vi "Read Control Height.vi"(8 "error in":errorcluster, 11 "Control in":refnum<vi>) -> (0 "error out":errorcluster, 2 "Height":u32, 3 "Control":refnum<vi>)   [LabVIEW 2020, in "VolatusGUIEditorCore.lvlib"]
uses:
  VolatusGUIEditorCore.lvlib
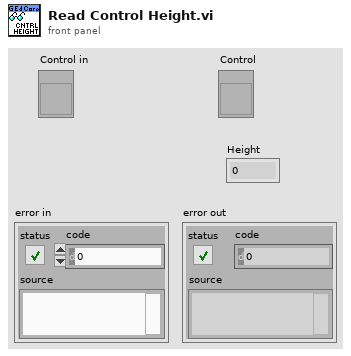
[diagram p1: front panel]
types:
  T1 = typedef "LVRectTypeDef.ctl" = cluster{"Left":i16, "Top":i16, "Right":i16, "Bottom":i16}
  T2 = typedef "LVBoundsTypeDef.ctl" = cluster{"Width":u32, "Height":u32}
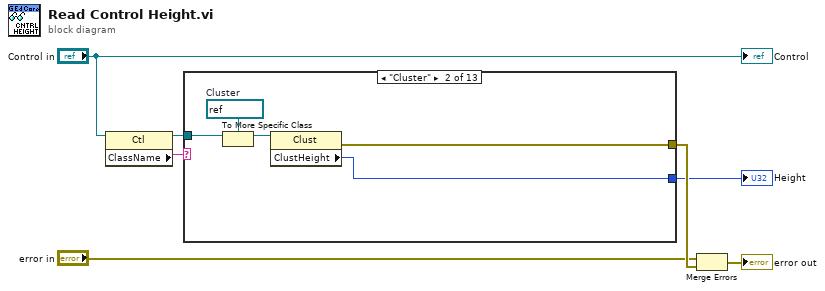
[diagram p0: block diagram]
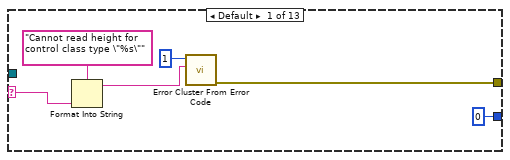
[diagram p2: hidden frame]
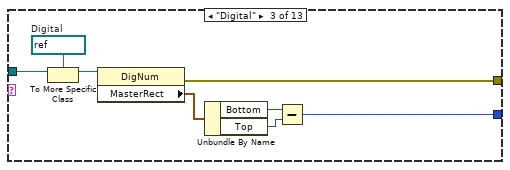
[diagram p3: hidden frame]
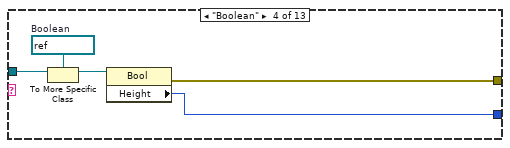
[diagram p4: hidden frame]
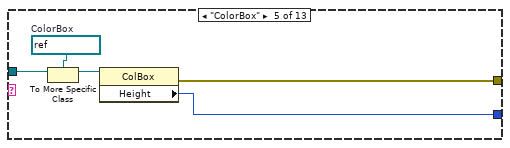
[diagram p5: hidden frame]
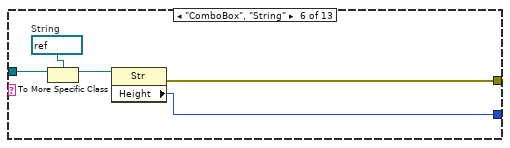
[diagram p6: hidden frame]
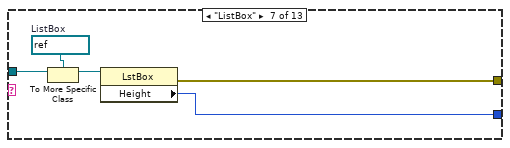
[diagram p7: hidden frame]
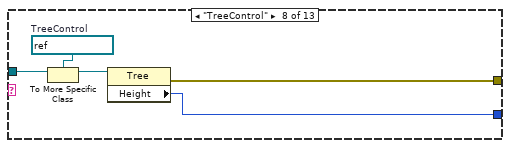
[diagram p8: hidden frame]
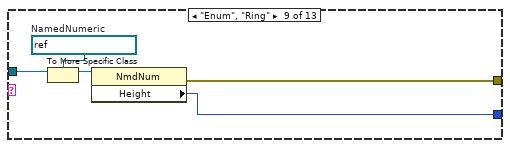
[diagram p9: hidden frame]
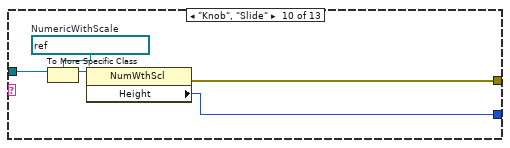
[diagram p10: hidden frame]
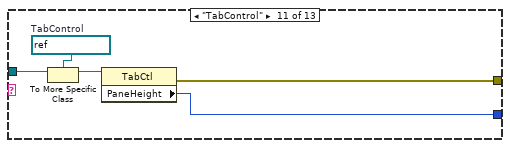
[diagram p11: hidden frame]
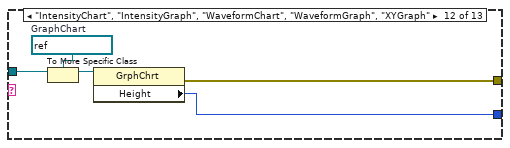
[diagram p12: hidden frame]
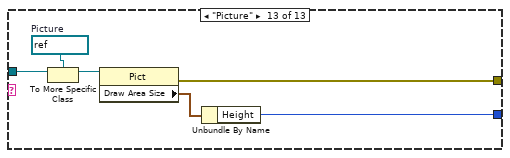
[diagram p13: hidden frame]
diagram:
  n1 = property class="Ctl"(reference="Control in") -> (reference out=w6:refnum<vi>, "ClassName"=w7:string)  [unwired: 1 in, 1 out]
  n2 = case shown="\"Cluster\"" w7 {
    selector: w7 -> [w10 _ _ _ _ _ _ _ _ _ _ _ _]
    tunnel: w6 -> [_ w18 w26 w31 w36 w41 w46 w51 w56 w61 w66 w71 w77]
    tunnel: [w13 w15 w23 w28 w33 w38 w43 w48 w53 w58 w63 w68 w74] -> w4
    tunnel: [u32 0 ("Height") w14 w19 w27 w32 w37 w42 w47 w52 w57 w62 w67 w72] -> w1
    frame Default {
      n3 = Format Into String(format string="Cannot read height for control class type \"%s\"", w10) -> (resulting string=w9:string)  [unwired: 2 in, 1 out]
      n4 = call <vilib>:"Error Cluster From Error Code.vi"("error message (\"\")"=w9, "error code (0)"=1) -> ("error out"=w13:errorcluster)  [unwired: 7 in]
    }
    frame "Cluster" {
      w17 = refnum<vi> refnum  # Cluster
      n5 = To More Specific Class(target class=w17, reference=w18) -> (specific class reference=w16:refnum<vi>)  [unwired: 1 in, 1 out]
      n6 = property class="Clust"(reference=w16) -> (error out=w15:errorcluster, "ClustHeight"=w14:u32)  [unwired: 1 in, 1 out]
    }
    frame "Digital" {
      w25 = refnum<vi> refnum  # Digital
      n7 = To More Specific Class(target class=w25, reference=w26) -> (specific class reference=w24:refnum<vi>)  [unwired: 1 in, 1 out]
      n8 = property class="DigNum"(reference=w24) -> (error out=w23:errorcluster, "MasterRect"=w22:T1)  [unwired: 1 in, 1 out]
      n9 = Unbundle By Name(w22) -> ("Bottom"=w21:i16, "Top"=w20:i16)
      n10 = Subtract(x=w21, y=w20) -> (x-y=w19:i16)
    }
    frame "Boolean" {
      w30 = refnum<vi> refnum  # Boolean
      n11 = To More Specific Class(target class=w30, reference=w31) -> (specific class reference=w29:refnum<vi>)  [unwired: 1 in, 1 out]
      n12 = property class="Bool"(reference=w29) -> (error out=w28:errorcluster, "Height"=w27:u32)  [unwired: 1 in, 1 out]
    }
    frame "ColorBox" {
      w35 = refnum<vi> refnum  # ColorBox
      n13 = To More Specific Class(target class=w35, reference=w36) -> (specific class reference=w34:refnum<vi>)  [unwired: 1 in, 1 out]
      n14 = property class="ColBox"(reference=w34) -> (error out=w33:errorcluster, "Height"=w32:u32)  [unwired: 1 in, 1 out]
    }
    frame "ComboBox", "String" {
      w40 = refnum<vi> refnum  # String
      n15 = To More Specific Class(target class=w40, reference=w41) -> (specific class reference=w39:refnum<vi>)  [unwired: 1 in, 1 out]
      n16 = property class="Str"(reference=w39) -> (error out=w38:errorcluster, "Height"=w37:u32)  [unwired: 1 in, 1 out]
    }
    frame "ListBox" {
      w45 = refnum<vi> refnum  # ListBox
      n17 = To More Specific Class(target class=w45, reference=w46) -> (specific class reference=w44:refnum<vi>)  [unwired: 1 in, 1 out]
      n18 = property class="LstBox"(reference=w44) -> (error out=w43:errorcluster, "Height"=w42:u32)  [unwired: 1 in, 1 out]
    }
    frame "TreeControl" {
      w50 = refnum<vi> refnum  # TreeControl
      n19 = To More Specific Class(target class=w50, reference=w51) -> (specific class reference=w49:refnum<vi>)  [unwired: 1 in, 1 out]
      n20 = property class="Tree"(reference=w49) -> (error out=w48:errorcluster, "Height"=w47:u32)  [unwired: 1 in, 1 out]
    }
    frame "Enum", "Ring" {
      w55 = refnum<vi> refnum  # NamedNumeric
      n21 = To More Specific Class(target class=w55, reference=w56) -> (specific class reference=w54:refnum<vi>)  [unwired: 1 in, 1 out]
      n22 = property class="NmdNum"(reference=w54) -> (error out=w53:errorcluster, "Height"=w52:u32)  [unwired: 1 in, 1 out]
    }
    frame "Knob", "Slide" {
      w60 = refnum<vi> refnum  # NumericWithScale
      n23 = To More Specific Class(target class=w60, reference=w61) -> (specific class reference=w59:refnum<vi>)  [unwired: 1 in, 1 out]
      n24 = property class="NumWthScl"(reference=w59) -> (error out=w58:errorcluster, "Height"=w57:u32)  [unwired: 1 in, 1 out]
    }
    frame "TabControl" {
      w65 = refnum<vi> refnum  # TabControl
      n25 = To More Specific Class(target class=w65, reference=w66) -> (specific class reference=w64:refnum<vi>)  [unwired: 1 in, 1 out]
      n26 = property class="TabCtl"(reference=w64) -> (error out=w63:errorcluster, "PaneHeight"=w62:u32)  [unwired: 1 in, 1 out]
    }
    frame "IntensityChart", "IntensityGraph", "WaveformChart", "WaveformGraph", "XYGraph" {
      w70 = refnum<vi> refnum  # GraphChart
      n27 = To More Specific Class(target class=w70, reference=w71) -> (specific class reference=w69:refnum<vi>)  [unwired: 1 in, 1 out]
      n28 = property class="GrphChrt"(reference=w69) -> (error out=w68:errorcluster, "Height"=w67:u32)  [unwired: 1 in, 1 out]
    }
    frame "Picture" {
      w76 = refnum<vi> refnum  # Picture
      n29 = To More Specific Class(target class=w76, reference=w77) -> (specific class reference=w75:refnum<vi>)  [unwired: 1 in, 1 out]
      n30 = property class="Pict"(reference=w75) -> (error out=w74:errorcluster, "Draw Area Size"=w73:T2)  [unwired: 1 in, 1 out]
      n31 = Unbundle By Name(w73) -> ("Height"=w72:u32)
    }
  }
  "Height" <- w1
  n32 = Merge Errors("error in", w4) -> (→"error out":errorcluster)
  "Control" <- "Control in"
